vi "Install All 1.0.vi"(7 "Restart Automatically (T)":bool=TRUE, 8 "error in (no error)":errorcluster, 10 "Deselect Conflicts (F)":bool, 11 "Session in":refnum<k21>) -> (0 "error out":errorcluster, 1 "Broken Dependencies":T1[](array[typedef]), 2 "Installed Software":T2[](array[typedef]), 3 "Session out":refnum<k21>)   [LabVIEW 2012, in "nisyscfg.lvlib"]
uses:
  <vilib>/nisyscfg/nisyscfg.lvlib
  <vilib>/nisyscfg/Software.ctl
  <vilib>/nisyscfg/Broken Dependency.ctl
  <vilib>/nisyscfg/Install All.vi
panel:
  # "This cluster is deprecated.\nUse Broken Dependency 1.2.ctl."
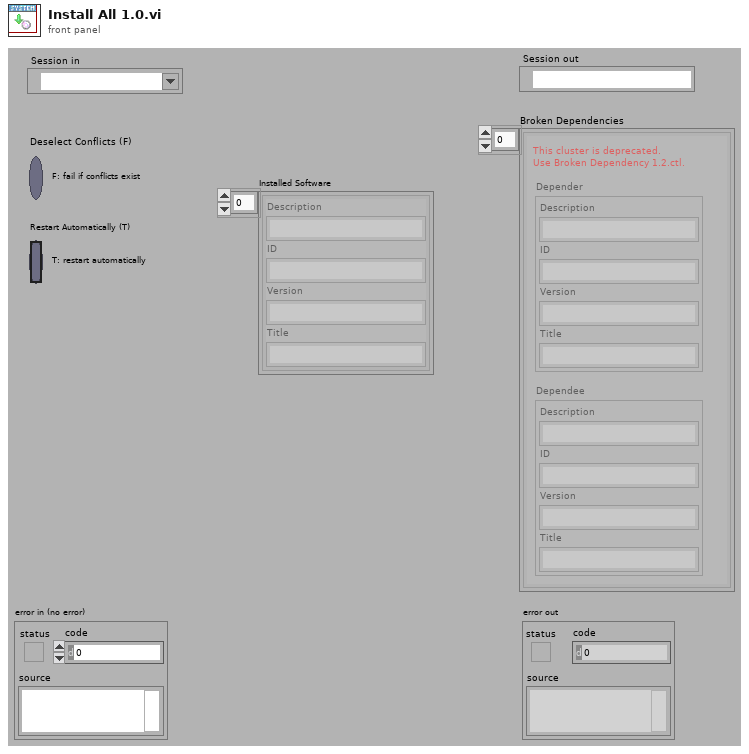
[diagram p1: front panel]
types:
  T1 = typedef "nisyscfg.lvlib/Broken Dependency.ctl" = cluster{"Depender":T2, "Dependee":T2}
  T2 = typedef "nisyscfg.lvlib/Software.ctl" = cluster{"Description":string, "ID":string, "Version":string, "Title":string}
  T3 = typedef "nisyscfg.lvlib/Broken Dependency 1.2.ctl" = cluster{"depender":T4, "dependee":T4}
  T4 = typedef "nisyscfg.lvlib/Software 1.2.ctl" = cluster{"title":string, "description":string, "ID":string, "version":string, "component type":T5}
  T5 = typedef "nisyscfg.lvlib/Component Type.ctl" = u32
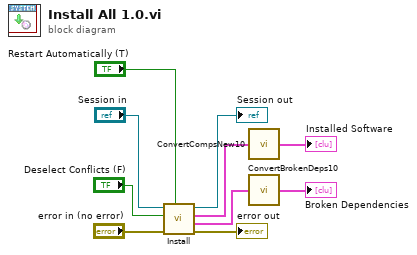
[diagram p0: block diagram]
diagram:
  n1 = call-poly <vilib>:"Install.vi"("Restart Automatically (T)"="Restart Automatically (T)", "error in (no error)"="error in (no error)", "Deselect Conflicts (F)"="Deselect Conflicts (F)", "Session in"="Session in") -> ("error out"=→"error out":errorcluster, "Broken Dependencies"=w2:T3[], "Installed Software"=w4:T4[], "Session out"=→"Session out":refnum<k21>)  [unwired: 4 in]
  n2 = call <vilib>:"ConvertCompsNew10.vi"("components 1.2"=w4) -> ("components 1.0"=→"Installed Software":T2[])
  n3 = call <vilib>:"ConvertBrokenDeps10.vi"("dependencies 1.2"=w2) -> ("dependencies 1.0"=→"Broken Dependencies":T1[])
